vi "AMX-CCD3 自动处理图像 - 副本.vi"(0 "Image IN":T1(plugin-control), 5 "Image Name1":string="Test2", 7 "Image Name2":string="Test3", 9 "A/B段位置切换":bool, 11 "error in (no error)":errorcluster caption="错误输入（无错误）", 12 "Image Name2 2":string="Test3") -> (4 "Image Out":T1(plugin-control), 6 "结果":bool, 10 "颗粒物有无判断":bool, 14 "结果数组":bool[](array[boolean]), 15 "error out":errorcluster caption="错误输出")   [LabVIEW 2017]
uses:
  Global System.vi
panel:
  out "Number of Features Found":i32
  in  "颗粒物个数阈值":i32
  out "颗粒物大小显示":dbl[](array[numeric])
  out "颗粒物位置坐标":cluster{"X":dbl, "Y":dbl}[](array[cluster]) {"Y" format="%.2f"; "X" format="%.2f"}
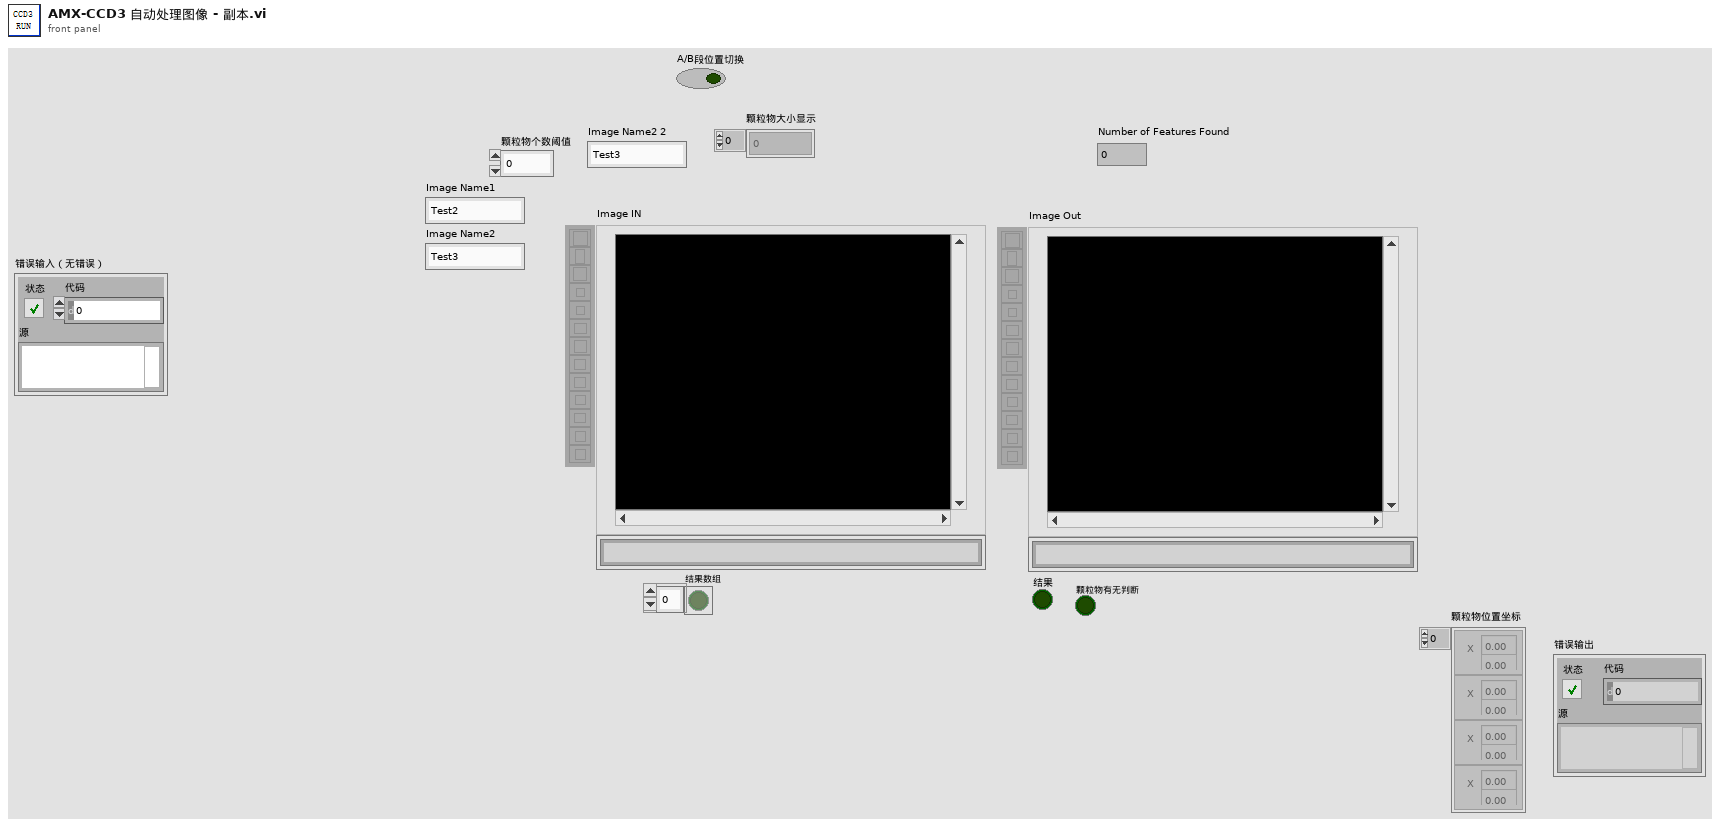
[diagram p1: front panel]
types:
  T1 = typedef "IMAQ Image.ctl" = refnum<image>
  T2 = cluster{"Desired Font (Application)":enum16{"User-specified Font", "Application Font", "System Font", "Dialog Font"}, "[User-specified Font]":cluster{"Font Name":string, "Size":i16, "Strikeout?":bool, "Italic?":bool, "Underline?":bool, "Outline?":bool, "Shadow?":bool, "Bold?":bool, "Rotation Angle":dbl}, "Horizontal Alignment":i16, "Vertical Alignment":i16}
  T3 = typedef "Image Type" = u32
  T4 = typedef "IMAQ Rectangle" = cluster{"Left":i32, "Top":i32, "Right":i32, "Bottom":i32, "Rotation":dbl}
  T5 = cluster{"Rectangle":T4, "Threshold Limits (Threshold 1)":cluster{"Lower value":sgl, "Upper value":sgl}, "Keep/Remove Particles ":bool, "Connectivity 4/8 (8) ":bool, "Selection Values (Particle Filter 1)":cluster{"Measurement Parameter":i32, "Range Lower Value":dbl, "Range Upper Value":dbl, "Range":bool, "Measurement Type":bool}[], "Corner Options (Feature Detection 1)":cluster{"Detector type":enum32{"Harris Corner", "Shi-Tomasi Corner"}, "Kernel size":i32, "Min Corner Point Strength":dbl}, "Pyramid level (Feature Detection 1)":u32, "Method ":i32, "Look For":u32, "Method 2":i32, "ROI Descriptor (Clamp (Rake) 1)":cluster{"Global Rectangle":i32[], "Contours":cluster{"ID":enum32{"External", "Internal"}, "Type":u32, "Coordinates":i32[]}[]}}
  T6 = typedef "IMAQ Curve Parameters.ctl" = cluster{"Extraction Mode":u32, "Edge Threshold":i32, "Edge Filter Size":u32, "Min Length":i32, "Row Search Step Size":i32, "Col Search Step Size":i32, "Max Endpoint Gap":i32, "Closed":bool, "Subpixel":bool}
  T7 = cluster{"Curve Extraction Settings ":T6, "Color Mode (Histogram 1)":u16, "Range (Threshold 1)":cluster{"Lower value":sgl, "Upper value":sgl}, "Clamp Settings (Max Clamp 1)":cluster{"Angle Range (+/-)":dbl, "Edge Polarity":cluster{"Start":u32, "End":u32}}, "Settings (Clamp (Rake) 1)":cluster{"Contrast":i32, "Filter width":i32, "Steepness":i32, "Subsampling Ratio":u32, "Show Search Area":bool, "Show Search Lines":bool, "Show Edges Found":bool, "Show Result":bool}, "直径设定":cluster{"Lower value":sgl, "Upper value":sgl}}
  T8 = typedef "IMAQdx.ctl" = refnum<k21>
  T9 = cluster{"IsNorImage":bool, "Exposure Values":u32, "ImagePath":path, "相机选择":T8}
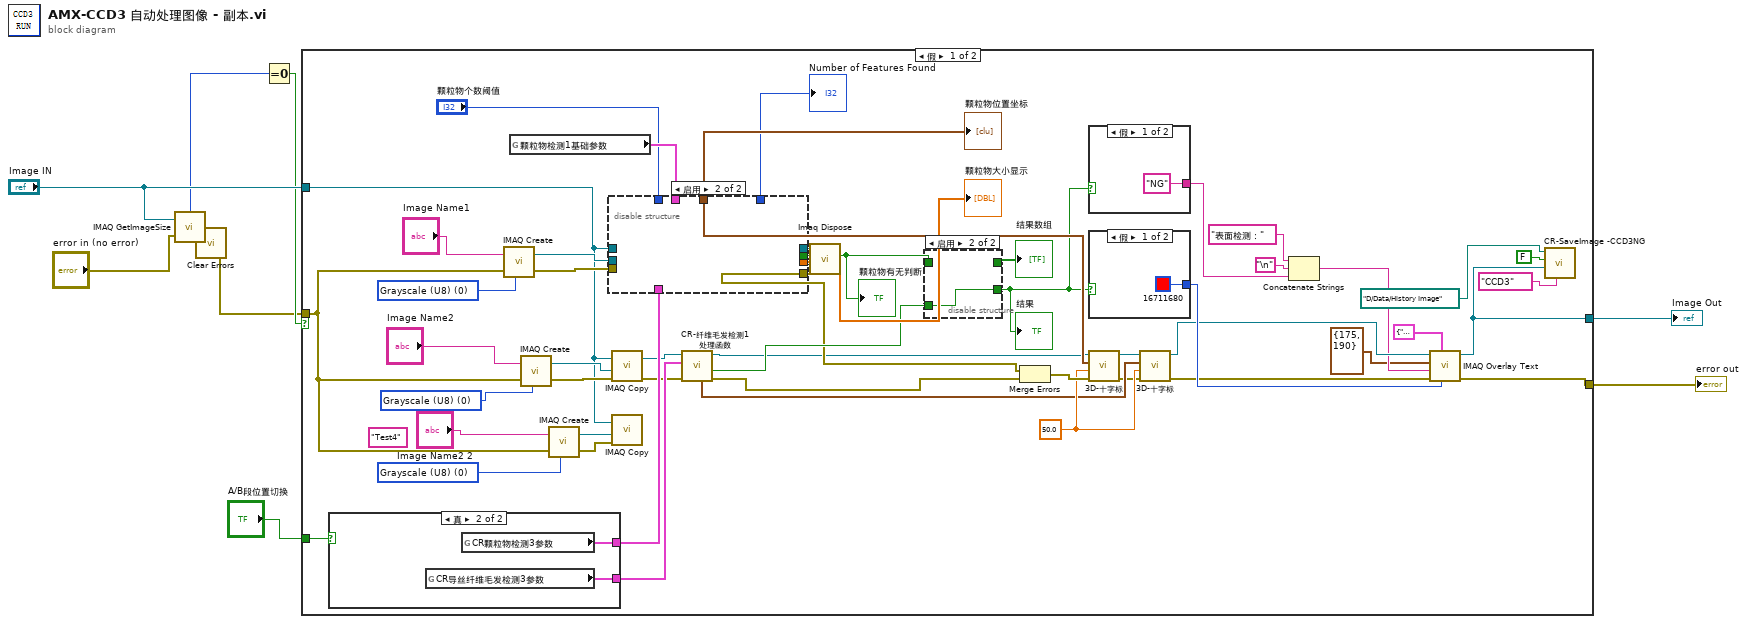
[diagram p0: block diagram]
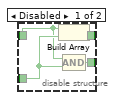
[diagram p2: hidden frame]
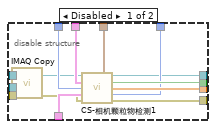
[diagram p3: hidden frame]
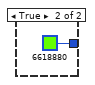
[diagram p4: hidden frame]
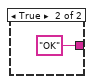
[diagram p5: hidden frame]
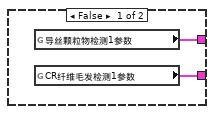
[diagram p6: hidden frame]
diagram:
  n1 = call "IMAQ GetImageSize"("Image"="Image IN", "error in (no error)"="error in (no error)") -> ("X Resolution"=w3:i32, "error out"=w4:errorcluster)  [unwired: 2 in, 1 out]
  n2 = call <vilib>:"Clear Errors.vi"("error in (no error)"=w4) -> ("error out"=w1:errorcluster)  [unwired: 5 in, 1 out]
  n3 = Equal To 0?(x=w3) -> (x = 0?=w2:bool)
  n4 = case shown="假" w2 {
    tunnel: "A/B段位置切换" -> [w60 _]
    tunnel: [w59 w88] -> w8
    tunnel: [w58 w89] -> w7
    tunnel: "Image IN" -> [w18 w89]
    tunnel: w1 -> [w17 w88]
    frame False {
      (unwired) "Test4" ("Image Name3")
      w12 = T3 0 items=["Grayscale (U8)", "Grayscale (I16)", "Grayscale (SGL)", "Complex (CSG)", "RGB (U32)", "HSL (U32)", "RGB (U64)", "Grayscale (U16)"] ("Image Type")
      w14 = T3 0 items=["Grayscale (U8)", "Grayscale (I16)", "Grayscale (SGL)", "Complex (CSG)", "RGB (U32)", "HSL (U32)", "RGB (U64)", "Grayscale (U16)"] ("Image Type")
      w16 = T3 0 items=["Grayscale (U8)", "Grayscale (I16)", "Grayscale (SGL)", "Complex (CSG)", "RGB (U32)", "HSL (U32)", "RGB (U64)", "Grayscale (U16)"] ("Image Type")
      w49 = 50.0 ("radius")
      n5 = case shown="真" w60 {
        tunnel: [w85 w87] -> w57
        tunnel: [w84 w86] -> w56
        frame False {
          n6 = global read "Global System.vi" "导丝颗粒物检测1参数"() -> (w85:T5)
          n7 = global read "Global System.vi" "CR纤维毛发检测1参数"() -> (w84:T7)
        }
        frame True {
          n8 = global read "Global System.vi" "CR导丝纤维毛发检测3参数"() -> (w86:T7)
          n9 = global read "Global System.vi" "CR颗粒物检测3参数"() -> (w87:T5)
        }
      }
      n10 = call "IMAQ Create"("Image Name"="Image Name1", "Image Type"=w14, "error in (no error)"=w17) -> ("New Image"=w24:T1, "error out"=w23:errorcluster)  [unwired: 2 in]
      n11 = global read "Global System.vi" "颗粒物检测1基础参数"() -> (w46:T9)
      n12 = call "IMAQ Create"("Image Name"="Image Name2", "Image Type"=w16, "error in (no error)"=w17) -> ("New Image"=w27:T1, "error out"=w30:errorcluster)  [unwired: 2 in]
      n13 = call "IMAQ Create"("Image Name"="Image Name2 2", "Image Type"=w12, "error in (no error)"=w17) -> ("New Image"=w20:T1, "error out"=w19:errorcluster)  [unwired: 2 in]
      n14 = disable-structure shown="启用" {
        disable-tunnel: w57 -> [w79 _]
        disable-tunnel: [w78 _] -> w54
        disable-tunnel: [w77 _] -> w51
        disable-tunnel: [w76 _] -> w50
        disable-tunnel: w46 -> [w75 _]
        disable-tunnel: [w74 _] -> w45
        disable-tunnel: [w73 _] -> w26
        disable-tunnel: "颗粒物个数阈值" -> [w72 _]
        disable-tunnel: w24 -> [w71 _]
        disable-tunnel: w23 -> [w69 _]
        disable-tunnel: [w67 _] -> w22
        disable-tunnel: w18 -> [w66 _]
        frame Disabled {
          n15 = call "IMAQ Copy"("error in (no error)"=w69, "Image Dst"=w71, "Image Src"=w66) -> ("error out"=w68:errorcluster, "Image Dst Out"=w70:T1)  [unwired: 3 in]
          n16 = call "CS-相机颗粒物检测1.vi"("Image in"=w70, "相机颗粒物检测1基础参数"=w75, "颗粒物个数阈值"=w72, "导丝颗粒物检测1参数"=w79, "error in (no error)"=w68) -> ("颗粒物位置坐标"=w77:cluster{"X":dbl, "Y":dbl}[], "Image out"=w73:T1, "颗粒物有无显示"=w76:bool, "颗粒物大小显示"=w78:dbl[], "Number of Features Found"=w74:i32, "error out"=w67:errorcluster)  [unwired: 4 in, 1 out]
        }
        frame Enabled {
        }
      }
      "颗粒物有无判断" <- w50
      "颗粒物位置坐标" <- w51
      "颗粒物大小显示" <- w54
      "Number of Features Found" <- w45
      n17 = call "IMAQ Copy"("error in (no error)"=w30, "Image Dst"=w27, "Image Src"=w18) -> ("error out"=w29:errorcluster, "Image Dst Out"=w28:T1)  [unwired: 3 in]
      n18 = call "IMAQ Copy"("error in (no error)"=w19, "Image Dst"=w20, "Image Src"=w18) -> ()  [unwired: 3 in, 2 out]
      n19 = call "CR-纤维毛发检测1处理函数.vi"("error in (no error)"=w29, "UI电源线正面漏线参数"=w56, "Image in"=w28) -> ("error out"=w21:errorcluster, "纤维毛发"=w53:bool, "Image out"=w10:T1, "Edge Coordinates (calibrated) (Clamp (Rake) 1)"=w48:cluster{"X":sgl, "Y":sgl}[])  [unwired: 4 in, 1 out]
      n20 = call "Imaq Dispose"("Image"=w26, "error in (no error)"=w22) -> ()  [unwired: 4 in, 1 out]
      n21 = disable-structure shown="启用" {
        disable-tunnel: [w64 _] -> w55
        disable-tunnel: w53 -> [w63 w65]
        disable-tunnel: w50 -> [w62 _]
        disable-tunnel: [w61 w65] -> w47
        frame Disabled {
          n22 = Build Array(w62, w63) -> (w64:bool[])
          n23 = Compound Arithmetic op=AND ("复合运算")(w62, w63) -> (w61:bool)
        }
        frame Enabled {
        }
      }
      "结果数组" <- w55
      "结果" <- w47
      n24 = Merge Errors(w22, w21) -> (w52:errorcluster)
      n25 = case shown="假" w47 {
        tunnel: ["NG" "OK"] -> w43
        frame False {
        }
        frame True {
        }
      }
      n26 = case shown="假" w47 {
        tunnel: [u32 16711680 ("Text Color (black)") u32 6618880 ("Text Color (black)")] -> w44
        frame False {
        }
        frame True {
        }
      }
      n27 = call "3D-十字标.vi"("error in (no error)"=w52, "radius"=w49, "颗粒物位置坐标"=w51, "输入图片"=w10) -> ("error out"=w39:errorcluster, "输出图片"=w40:T1)  [unwired: 6 in]
      n28 = call "3D-十字标.vi"("error in (no error)"=w39, "radius"=w49, "颗粒物位置坐标"=w48, "输入图片"=w40) -> ("error out"=w41:errorcluster, "输出图片"=w42:T1)  [unwired: 6 in]
      n29 = Concatenate Strings("表面检测：" ("字符串"), "\n", w43) -> (w35:string)
      n30 = call "IMAQ Overlay Text"("Text Color (black)"=w44, "Font, Size & Style"=T2 {"Desired Font (Application)"=enum."User-specified Font", "[User-specified Font]"={"Font Name"="", "Size"=100, "Strikeout?"=FALSE, "Italic?"=FALSE, "Underline?"=FALSE, "Outline?"=FALSE, "Shadow?"=FALSE, "Bold?"=FALSE, "Rotation Angle"=0.0}, "Horizontal Alignment"=0, "Vertical Alignment"=0}, "error in (no error)"=w41, "String"=w35, "Origin"=cluster{"X":i32, "Y":i32} {"X"=175, "Y"=190}, "Image"=w42) -> ("error out"=w59:errorcluster, "Image Out"=w58:T1)  [unwired: 4 in]
      n31 = call "CR-SaveImage -CCD3NG.vi"("CCD Name"="CCD3", "Image in"=w58, "布尔"=FALSE, "基路径"=path "D:/Data/History Image") -> ()  [unwired: 7 in, 1 out]
    }
    frame True {
    }
  }
  "error out" <- w8
  "Image Out" <- w7
